vi "Delete_Overlay_2Images-1.vi"(3 "error IN":errorcluster, 4 "2nd Image IN":T1, 5 "1st Image IN":T1, 6 "Delete \nOverlay?":bool) -> (0 "error OUT":errorcluster, 1 "2nd Image OUT":T1, 2 "1st Image OUT":T1)   [LabVIEW 2013]
uses:
  <vilib>/vision/Image Controls.llb/IMAQ Image.ctl
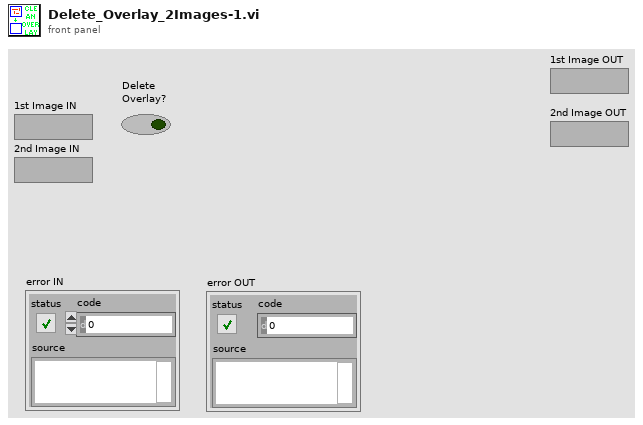
[diagram p1: front panel]
types:
  T1 = typedef "IMAQ Image.ctl" = refnum<image>
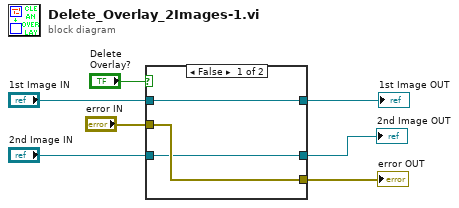
[diagram p0: block diagram]
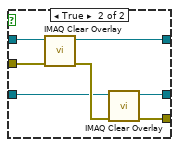
[diagram p2: hidden frame]
diagram:
  n1 = case shown="False" "Delete \nOverlay?" {
    tunnel: "1st Image IN" -> [w9 w17]
    tunnel: [w9 w15] -> w5
    tunnel: "error IN" -> [w10 w16]
    tunnel: [w8 w14] -> w1
    tunnel: [w10 w12] -> w3
    tunnel: "2nd Image IN" -> [w8 w11]
    frame False {
    }
    frame True {
      n2 = call "IMAQ Clear Overlay"("error in (no error)"=w16, "Image"=w17) -> ("error out"=w13:errorcluster, "Image Out"=w15:T1)  [unwired: 8 in]
      n3 = call "IMAQ Clear Overlay"("error in (no error)"=w13, "Image"=w11) -> ("error out"=w12:errorcluster, "Image Out"=w14:T1)  [unwired: 8 in]
    }
  }
  "1st Image OUT" <- w5
  "error OUT" <- w3
  "2nd Image OUT" <- w1
